vi "ReinitializeWhenStopped.vi"(11 "JoystickValue":dbl) -> (3 "reinitialize? (F)":bool)   [LabVIEW 2014]
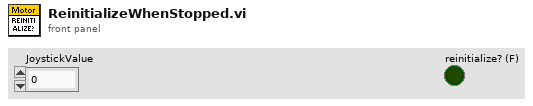
[diagram p1: front panel]
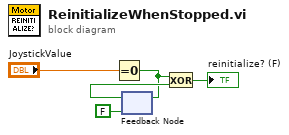
[diagram p0: block diagram]
diagram:
  n1 = Equal To 0?(x="JoystickValue") -> (x = 0?=w2:bool)
  n2 = feedback-in #1(w2) -> ()
  n3 = feedback #1(FALSE) -> (w3:bool)
  n4 = Exclusive Or(1:w3, 2:w2) -> (0:→"reinitialize? (F)":bool)
